vi "Write Test Sequences.vi"(8 "error in (no error)":errorcluster, 10 "Test Sequences":T2(array[cluster]), 11 "CK in":refnum<class "CK.lvclass">) -> (0 "error out":errorcluster, 3 "CK out":refnum<class "CK.lvclass">)   [LabVIEW 2020, in "CK.lvclass"]
uses:
  CK.lvclass
  Controls/Register to Write.ctl
  CK.lvclass/CK.ctl
  PIC-device/PIC-Device.lvclass
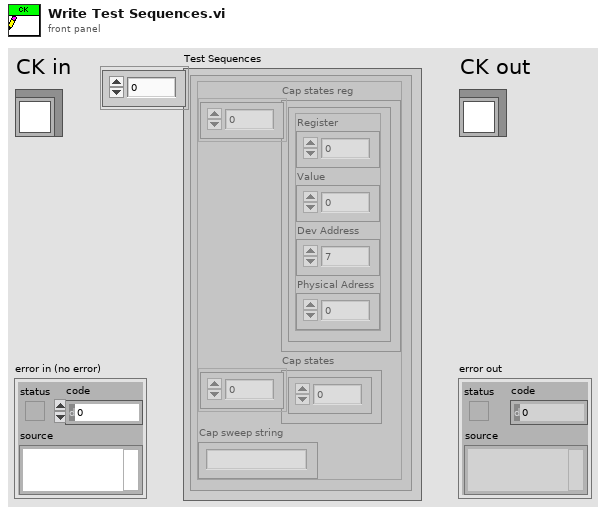
[diagram p1: front panel]
types:
  T1 = typedef "PIC-Device.lvclass/Register to Write.ctl" = cluster{"Register":u32, "Value":u32, "Dev Address":u32, "Physical Adress":u32}
  T2 = cluster{"Cap states reg":T1[], "Cap states":dbl[], "Cap sweep string":string}[]
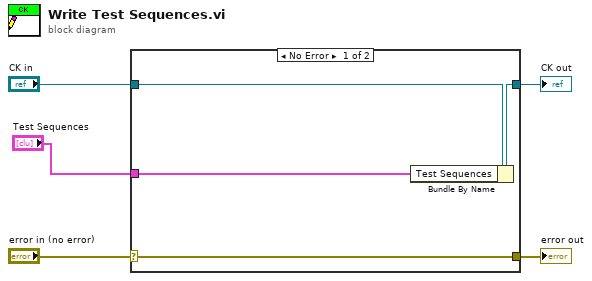
[diagram p0: block diagram]
diagram:
  n1 = case shown="No Error" "error in (no error)" {
    selector: "error in (no error)" -> [w9 w10]
    tunnel: [w9 w10] -> w4
    tunnel: [w7 w11] -> w2
    tunnel: "CK in" -> [w8 w11]
    tunnel: "Test Sequences" -> [w6 _]
    frame No Error {
      n2 = Bundle By Name(cluster=w8, "Test Sequences"=w6) -> (w7:refnum<class "CK.lvclass">)
    }
    frame Error {
    }
  }
  "error out" <- w4
  "CK out" <- w2
